vi "joysticksLoop.vi"(8 "Second JoystickDevRef":T1, 9 "Main JoystickDevRef":T1={"Device"=enum."USB 1"}) -> ()   [LabVIEW 2018]
doc: "This VI is called for each TeleOp packet received from the DS where the robot is not disabled. It is often used to read from the joysticks and update I/O or to update setpoints for timed control loops. It should complete and return within 20 milliseconds or it may miss DS packets."
uses:
  <vilib>/Rock Robotics/WPI/Joystick/WPI_JoystickDevRef.ctl
  <vilib>/Rock Robotics/WPI/Joystick/WPI_JoystickDeviceEnum.ctl
  <vilib>/Platform/TimedLoop/XDataNode/timing_clust.ctl
  <vilib>/Platform/TimedLoop/XDataNode/nitl_modes.ctl
  <vilib>/Platform/TimedLoop/XDataNode/wakeup.ctl
  <vilib>/platform/TimedLoop/XDataNode/XDataNode.xnode
  <vilib>/Platform/TimedLoop/XDataNode/XDNodeRunTimeDep.lvlib
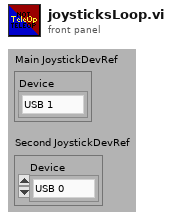
[diagram p1: front panel]
types:
  T1 = typedef "WPI_JoystickDevRef.ctl" = cluster{"Device":T2}
  T2 = typedef "WPI_JoystickDeviceEnum.ctl" = enum16{"USB 0", "USB 1", "USB 2", "USB 3", "USB 4", "USB 5"}
  T3 = typedef "XDNodeRunTimeDep.lvlib/timing_clust.ctl" = cluster{"Expected End [f-1]":u64, "Actual End [f-1]":u64, "Finished Late? [f-1]":bool, "Expected End [i-1]":u64, "Actual End [i-1]":u64, "Finished Late? [i-1]":bool, "Expected Start [i]":u64, "Actual Start [i]":u64, "Expected Start [f]":u64, "Actual Start [f]":u64, "Source Name":string, "Structure Name":string, "Period":i64, "Deadline":i64, "Offset":i64, "Start":i64, "Priority":i32, "Timeout":i32, "Mode":T4, "Wakeup Reason":T5, "Error":errorcluster, "Source Type":string, "Secondary Source Type":string, "Global End Time":u64, "Global Start Time":u64, "Frame Duration":u64, "Iteration Duration":u64, "Assigned CPU":i32, "I/O Scan Engine Mode":u32}
  T4 = typedef "XDNodeRunTimeDep.lvlib/nitl_modes.ctl" = enum32{"No Change", "Process missed periods, maintain original phase", "Discard missed periods, maintain original phase", "Process missed periods, ignore original phase", "Discard missed periods, ignore original phase"}
  T5 = typedef "XDNodeRunTimeDep.lvlib/wakeup.ctl" = enum32{"Normal", "Aborted", "Asynchronous wakeup", "Timing source error", "Timed loop error", "Timeout"}
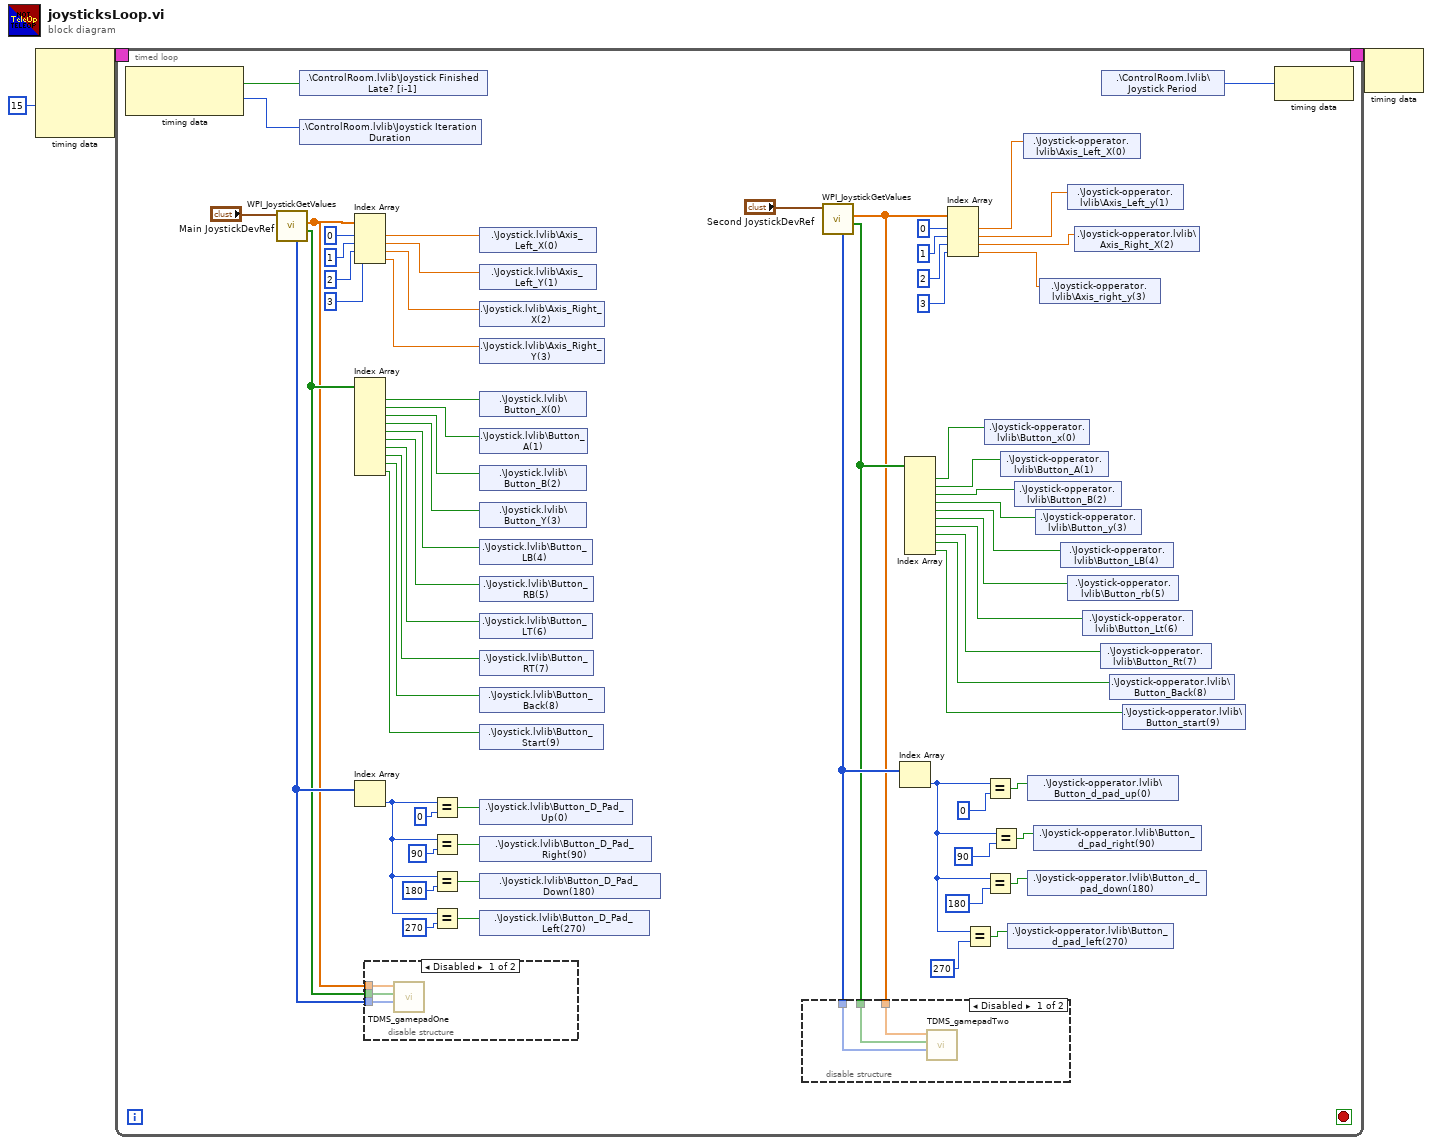
[diagram p0: block diagram]
diagram:
  n1 = node-c288(15 ("Priority")) -> (w3:T3)  [unwired: 3 in]
  n2 = timed-loop {
    timing: w3 -> [_]
    timing-out: [_] -> w2
    stop <- _ stop-if-true
    n3 = node-c288() -> (w6:bool, w5:i64)  [unwired: 1 in]
    n4 = call <vilib>:"WPI_JoystickGetValues.vi"("JoystickDevRef"="Main JoystickDevRef") -> ("Buttons"=w40:bool[], "Axes"=w39:dbl[], "POVs"=w41:i16[])  [unwired: 6 in, 2 out]
    n5 = shared-variable ".\\ControlRoom.lvlib\\Joystick Finished Late? [i-1]"(w6) -> ()  [unwired: 1 in, 1 out]
    n6 = shared-variable ".\\ControlRoom.lvlib\\Joystick Iteration Duration"(w5) -> ()  [unwired: 1 in, 1 out]
    n7 = Index Array(array=w39, index #1=0 ("index"), index #2=1 ("index"), index #3=2 ("index"), index #4=3 ("index")) -> (element #1=w68:dbl, element #2=w65:dbl, element #3=w66:dbl, element #4=w67:dbl)
    n8 = Index Array(array=w40) -> (element #1=w64:bool, element #2=w63:bool, element #3=w62:bool, element #4=w61:bool, element #5=w60:bool, element #6=w42:bool, element #7=w59:bool, element #8=w58:bool, element #9=w57:bool, element #10=w56:bool)  [unwired: 10 in]
    n9 = Index Array(array=w41) -> (element=w51:i16)  [unwired: 1 in]
    n10 = disable-structure shown="Disabled" {
      disable-tunnel: w41 -> [w74 _]
      disable-tunnel: w40 -> [w73 _]
      disable-tunnel: w39 -> [w72 _]
      frame Disabled {
        n11 = call "TDMS_gamepadOne.vi"("POVs"=w74, "Buttons"=w73, "Axes"=w72) -> ()  [unwired: 9 in]
      }
      frame Enabled {
      }
    }
    n12 = Equal?(x=w51, y=i16 0) -> (x = y?=w50:bool)
    n13 = Equal?(x=w51, y=i16 90) -> (x = y?=w47:bool)
    n14 = Equal?(x=w51, y=i16 180) -> (x = y?=w48:bool)
    n15 = Equal?(x=w51, y=i16 270) -> (x = y?=w49:bool)
    n16 = shared-variable ".\\Joystick.lvlib\\Axis_Left_X(0)"(w68) -> ()  [unwired: 1 in, 1 out]
    n17 = shared-variable ".\\Joystick.lvlib\\Axis_Left_Y(1)"(w65) -> ()  [unwired: 1 in, 1 out]
    n18 = shared-variable ".\\Joystick.lvlib\\Axis_Right_X(2)"(w66) -> ()  [unwired: 1 in, 1 out]
    n19 = shared-variable ".\\Joystick.lvlib\\Axis_Right_Y(3)"(w67) -> ()  [unwired: 1 in, 1 out]
    n20 = shared-variable ".\\Joystick.lvlib\\Button_X(0)"(w64) -> ()  [unwired: 1 in, 1 out]
    n21 = shared-variable ".\\Joystick.lvlib\\Button_A(1)"(w63) -> ()  [unwired: 1 in, 1 out]
    n22 = shared-variable ".\\Joystick.lvlib\\Button_B(2)"(w62) -> ()  [unwired: 1 in, 1 out]
    n23 = shared-variable ".\\Joystick.lvlib\\Button_Y(3)"(w61) -> ()  [unwired: 1 in, 1 out]
    n24 = shared-variable ".\\Joystick.lvlib\\Button_LB(4)"(w60) -> ()  [unwired: 1 in, 1 out]
    n25 = shared-variable ".\\Joystick.lvlib\\Button_RB(5)"(w42) -> ()  [unwired: 1 in, 1 out]
    n26 = shared-variable ".\\Joystick.lvlib\\Button_LT(6)"(w59) -> ()  [unwired: 1 in, 1 out]
    n27 = shared-variable ".\\Joystick.lvlib\\Button_RT(7)"(w58) -> ()  [unwired: 1 in, 1 out]
    n28 = shared-variable ".\\Joystick.lvlib\\Button_Back(8)"(w57) -> ()  [unwired: 1 in, 1 out]
    n29 = shared-variable ".\\Joystick.lvlib\\Button_Start(9)"(w56) -> ()  [unwired: 1 in, 1 out]
    n30 = shared-variable ".\\Joystick.lvlib\\Button_D_Pad_Up(0)"(w50) -> ()  [unwired: 1 in, 1 out]
    n31 = shared-variable ".\\Joystick.lvlib\\Button_D_Pad_Right(90)"(w47) -> ()  [unwired: 1 in, 1 out]
    n32 = shared-variable ".\\Joystick.lvlib\\Button_D_Pad_Down(180)"(w48) -> ()  [unwired: 1 in, 1 out]
    n33 = shared-variable ".\\Joystick.lvlib\\Button_D_Pad_Left(270)"(w49) -> ()  [unwired: 1 in, 1 out]
    n34 = call <vilib>:"WPI_JoystickGetValues.vi"("JoystickDevRef"="Second JoystickDevRef") -> ("Buttons"=w10:bool[], "Axes"=w9:dbl[], "POVs"=w11:i16[])  [unwired: 6 in, 2 out]
    n35 = disable-structure shown="Disabled" {
      disable-tunnel: w11 -> [w71 _]
      disable-tunnel: w10 -> [w70 _]
      disable-tunnel: w9 -> [w69 _]
      frame Disabled {
        n36 = call "TDMS_gamepadTwo.vi"("POVs"=w71, "Buttons"=w70, "Axes"=w69) -> ()  [unwired: 9 in]
      }
      frame Enabled {
      }
    }
    n37 = Index Array(array=w11) -> (element=w20:i16)  [unwired: 1 in]
    n38 = Index Array(array=w10) -> (element #1=w33:bool, element #2=w29:bool, element #3=w28:bool, element #4=w27:bool, element #5=w26:bool, element #6=w25:bool, element #7=w24:bool, element #8=w23:bool, element #9=w22:bool, element #10=w21:bool)  [unwired: 10 in]
    n39 = Index Array(array=w9, index #1=0 ("index"), index #2=1 ("index"), index #3=2 ("index"), index #4=3 ("index")) -> (element #1=w34:dbl, element #2=w32:dbl, element #3=w31:dbl, element #4=w30:dbl)
    n40 = Equal?(x=w20, y=i16 270) -> (x = y?=w12:bool)
    n41 = shared-variable ".\\Joystick-opperator.lvlib\\Button_x(0)"(w33) -> ()  [unwired: 1 in, 1 out]
    n42 = Equal?(x=w20, y=i16 0) -> (x = y?=w15:bool)
    n43 = Equal?(x=w20, y=i16 180) -> (x = y?=w13:bool)
    n44 = Equal?(x=w20, y=i16 90) -> (x = y?=w14:bool)
    n45 = shared-variable ".\\Joystick-opperator.lvlib\\Button_A(1)"(w29) -> ()  [unwired: 1 in, 1 out]
    n46 = shared-variable ".\\Joystick-opperator.lvlib\\Button_d_pad_left(270)"(w12) -> ()  [unwired: 1 in, 1 out]
    n47 = shared-variable ".\\Joystick-opperator.lvlib\\Button_B(2)"(w28) -> ()  [unwired: 1 in, 1 out]
    n48 = shared-variable ".\\Joystick-opperator.lvlib\\Axis_Left_X(0)"(w34) -> ()  [unwired: 1 in, 1 out]
    n49 = shared-variable ".\\Joystick-opperator.lvlib\\Button_d_pad_up(0)"(w15) -> ()  [unwired: 1 in, 1 out]
    n50 = shared-variable ".\\Joystick-opperator.lvlib\\Button_d_pad_down(180)"(w13) -> ()  [unwired: 1 in, 1 out]
    n51 = shared-variable ".\\Joystick-opperator.lvlib\\Button_d_pad_right(90)"(w14) -> ()  [unwired: 1 in, 1 out]
    n52 = shared-variable ".\\Joystick-opperator.lvlib\\Button_y(3)"(w27) -> ()  [unwired: 1 in, 1 out]
    n53 = shared-variable ".\\Joystick-opperator.lvlib\\Axis_right_y(3)"(w30) -> ()  [unwired: 1 in, 1 out]
    n54 = shared-variable ".\\Joystick-opperator.lvlib\\Button_LB(4)"(w26) -> ()  [unwired: 1 in, 1 out]
    n55 = shared-variable ".\\Joystick-opperator.lvlib\\Axis_Left_y(1)"(w32) -> ()  [unwired: 1 in, 1 out]
    n56 = shared-variable ".\\Joystick-opperator.lvlib\\Button_rb(5)"(w25) -> ()  [unwired: 1 in, 1 out]
    n57 = shared-variable ".\\Joystick-opperator.lvlib\\Axis_Right_X(2)"(w31) -> ()  [unwired: 1 in, 1 out]
    n58 = shared-variable ".\\Joystick-opperator.lvlib\\Button_Lt(6)"(w24) -> ()  [unwired: 1 in, 1 out]
    n59 = shared-variable ".\\Joystick-opperator.lvlib\\Button_Rt(7)"(w23) -> ()  [unwired: 1 in, 1 out]
    n60 = shared-variable ".\\ControlRoom.lvlib\\Joystick Period"() -> (w4:i64)  [unwired: 1 in, 1 out]
    n61 = shared-variable ".\\Joystick-opperator.lvlib\\Button_Back(8)"(w22) -> ()  [unwired: 1 in, 1 out]
    n62 = shared-variable ".\\Joystick-opperator.lvlib\\Button_start(9)"(w21) -> ()  [unwired: 1 in, 1 out]
    n63 = node-c288(w4) -> ()  [unwired: 1 out]
  }
  n64 = node-c288(w2) -> ()  [unwired: 1 out]
